vi "isclickinwindow.vi"(6 "Image Param":T1, 7 "Point32":T2) -> (0 "4 Y":i32, 1 "3 Height":i32, 2 "2 X":i32, 3 "1 Width":i32, 4 "In image?":bool)   [LabVIEW 2014]
uses:
  <vilib>/Utility/miscctls.llb/LVPoint32TypeDef.ctl
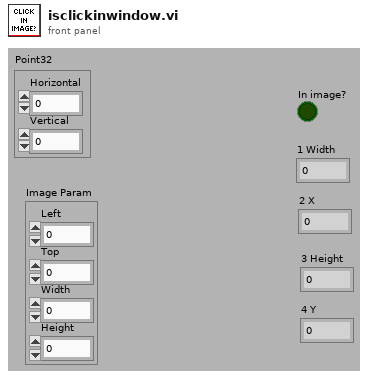
[diagram p1: front panel]
types:
  T1 = cluster{"Left":i32, "Top":i32, "Width":u32, "Height":u32}
  T2 = typedef "LVPoint32TypeDef.ctl" = cluster{"Horizontal":i32, "Vertical":i32}
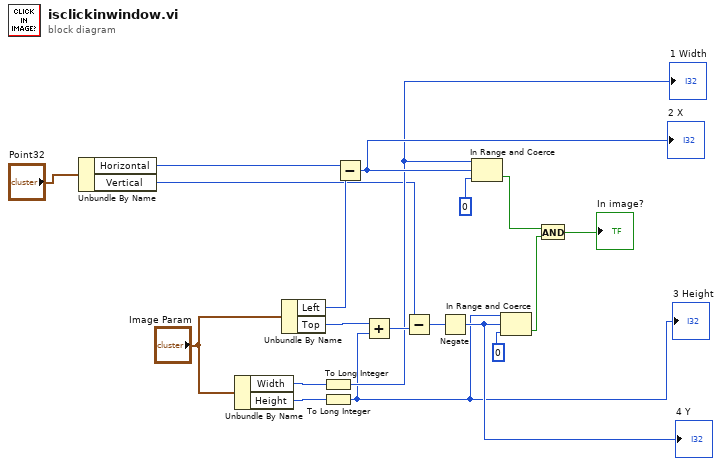
[diagram p0: block diagram]
diagram:
  n1 = Unbundle By Name("Point32") -> ("Horizontal"=w5:i32, "Vertical"=w4:i32)
  n2 = Unbundle By Name("Image Param") -> ("Width"=w3:u32, "Height"=w2:u32)
  n3 = Unbundle By Name("Image Param") -> ("Left"=w19:i32, "Top"=w18:i32)
  n4 = To Long Integer(number=w3) -> (32bit integer=w11:i32)
  "1 Width" <- w11
  n5 = To Long Integer(number=w2) -> (32bit integer=w10:i32)
  "3 Height" <- w10
  n6 = Subtract(x=w5, y=w19) -> (x-y=w15:i32)
  "2 X" <- w15
  n7 = Add(x=w18, y=w10) -> (x+y=w17:i32)
  n8 = Subtract(x=w4, y=w17) -> (x-y=w16:i32)
  n9 = Negate(x=w16) -> (-x=w14:i32)
  "4 Y" <- w14
  n10 = In Range and Coerce(upper limit=w11, x=w15, lower limit=0) -> (In Range?=w9:bool)  [unwired: 1 out]
  n11 = In Range and Coerce(upper limit=w10, x=w14, lower limit=0) -> (In Range?=w8:bool)  [unwired: 1 out]
  n12 = And(x=w9, y=w8) -> (x .and. y?=→"In image?":bool)
